vi "motion_server.vi"() -> ()   [LabVIEW 2012]
uses:
  motion_command.ctl
  motion_status.ctl
  <vilib>/Platform/TimedLoop/XDataNode/timing_clust.ctl
  <vilib>/Platform/TimedLoop/XDataNode/nitl_modes.ctl
  <vilib>/Platform/TimedLoop/XDataNode/wakeup.ctl
  <vilib>/Motion/FlexMotion/FunctionsVIs/StartStopMotion.llb/Stop Motion (6 axes).flx
  <vilib>/Platform/TimedLoop/XDataNode/XDataNode.xnode
  <vilib>/Platform/TimedLoop/XDataNode/XDNodeRunTimeDep.lvlib
panel:
  out "Home position":dbl[](array[numeric])
  out "End transform":dbl[](array[numeric])
  in  "Home":bool
  out "Motion status":T1={"Axis names"=["X", "Y", "Z", "Rx", "Ry", "Rz"], "Axis positions"=[], "Pose"=[], "Timestamp"=0, "Ready"=FALSE, "Stopped"=FALSE} {"Pose" format="%#.4f"; "Axis positions" format="%#.4f"}
  out "Stopped":bool
  in  "Emergency stop":bool
  in  "Home found":bool
  out "Command":T2={"Position"=[0.0, 0.0, 0.0, 0.0, 0.0, 0.0], "Axis enable"=[TRUE, TRUE, TRUE, TRUE, TRUE, TRUE], "Mode"=enum."Absolute axis", "Timestamp"=0}
  in  "Set origin":bool
  in  "stop":bool
  # "Motion server"
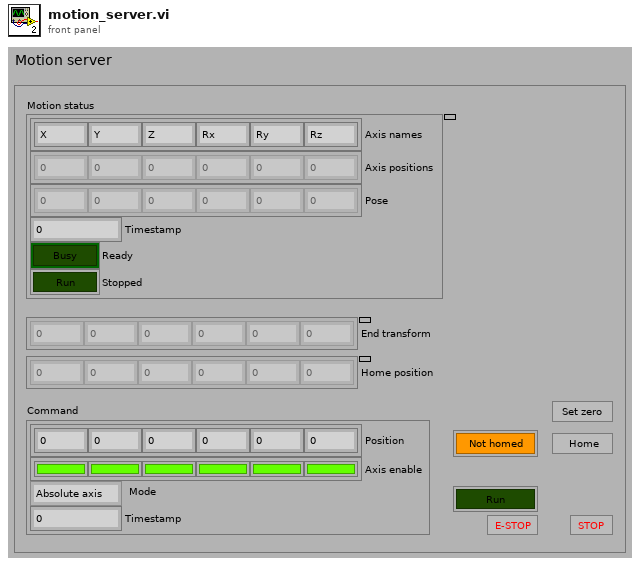
[diagram p1: front panel]
types:
  T1 = typedef "motion_status.ctl" = cluster{"Axis names":string[], "Axis positions":dbl[], "Pose":dbl[], "Timestamp":u32, "Ready":bool, "Stopped":bool}
  T2 = typedef "motion_command.ctl" = cluster{"Position":dbl[], "Axis enable":bool[], "Mode":enum16{"Absolute axis", "Relative axis", "Pose"}, "Timestamp":u32}
  T3 = typedef "Board Id" = u8
  T4 = typedef "Axis #" = cluster{"1":bool, "2":bool, "3":bool, "4":bool, "5":bool, "6":bool}
  T5 = typedef "XDNodeRunTimeDep.lvlib/timing_clust.ctl" = cluster{"Expected End [f-1]":u64, "Actual End [f-1]":u64, "Finished Late? [f-1]":bool, "Expected End [i-1]":u64, "Actual End [i-1]":u64, "Finished Late? [i-1]":bool, "Expected Start [i]":u64, "Actual Start [i]":u64, "Expected Start [f]":u64, "Actual Start [f]":u64, "Source Name":string, "Structure Name":string, "Period":i64, "Deadline":i64, "Offset":i64, "Start":i64, "Priority":i32, "Timeout":i32, "Mode":T6, "Wakeup Reason":T7, "Error":errorcluster, "Source Type":string, "Secondary Source Type":string, "Global End Time":u64, "Global Start Time":u64, "Frame Duration":u64, "Iteration Duration":u64, "Assigned CPU":i32, "I/O Scan Engine Mode":u32}
  T6 = typedef "XDNodeRunTimeDep.lvlib/nitl_modes.ctl" = enum32{"No Change", "Process missed periods, maintain original phase", "Discard missed periods, maintain original phase", "Process missed periods, ignore original phase", "Discard missed periods, ignore original phase"}
  T7 = typedef "XDNodeRunTimeDep.lvlib/wakeup.ctl" = enum32{"Normal", "Aborted", "Asynchronous wakeup", "Timing source error", "Timed loop error", "Timeout"}
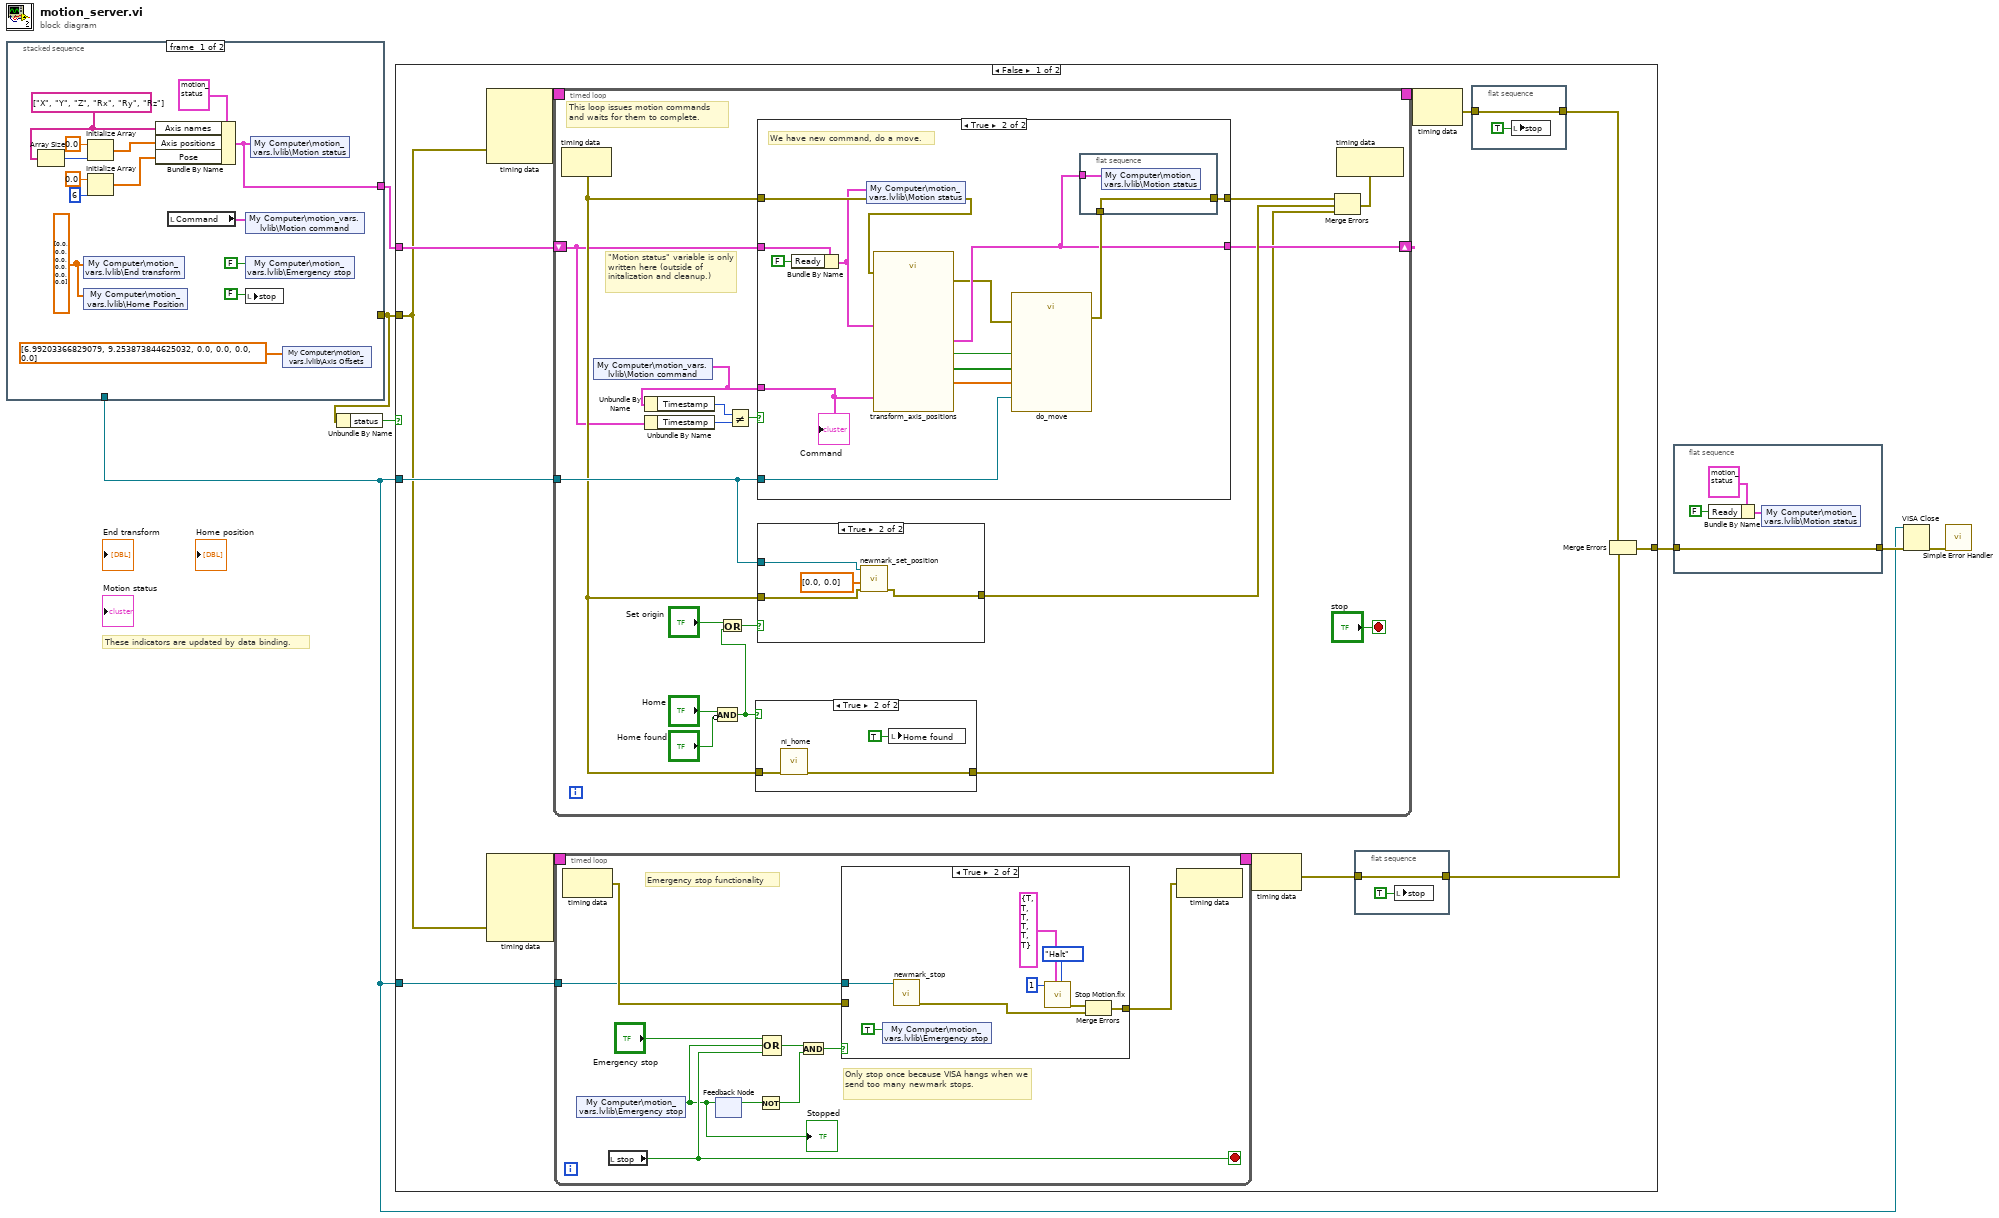
[diagram p0: block diagram]
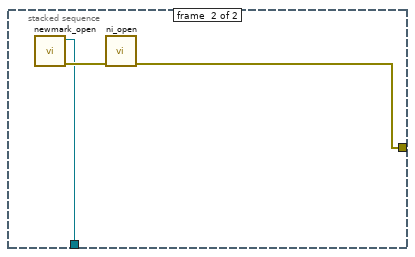
[diagram p2: hidden frame]
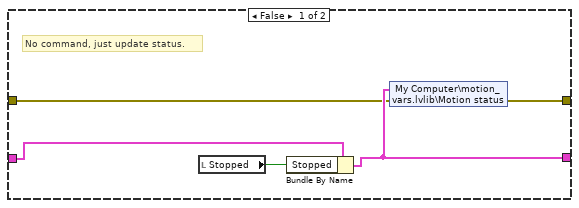
[diagram p6: hidden frame]
diagram:
  # "These indicators are updated by data binding."
  n1 = stacked-sequence {
    tunnel: [_ w22] -> w2
    tunnel: [w10 _] -> w3
    tunnel: [_ w23] -> w1
    frame #0 {
      w11 = string[] ["X", "Y", "Z", "Rx", "Ry", "Rz"] ("Axis names")
      w9 = dbl[] [0.0, 0.0, 0.0, 0.0, 0.0, 0.0] ("End transform")
      n2 = Array Size(array=w11) -> (size(s)=w19:i32)
      n3 = shared-variable "My Computer\\motion_vars.lvlib\\End transform"(w9) -> ()  [unwired: 1 in, 1 out]
      n4 = shared-variable "My Computer\\motion_vars.lvlib\\Home Position"(w9) -> ()  [unwired: 1 in, 1 out]
      n5 = Initialize Array(0.0, w19) -> (w17:dbl[])
      n6 = Initialize Array(0.0, 6 ("dimension size")) -> (w14:dbl[])
      n7 = Bundle By Name(cluster=T1 {"Axis names"=["X", "Y", "Z", "Rx", "Ry", "Rz"], "Axis positions"=[], "Pose"=[], "Timestamp"=0, "Ready"=TRUE, "Stopped"=FALSE} ("Motion status"), "Axis names"=w11, "Axis positions"=w17, "Pose"=w14) -> (w10:T1)
      n8 = local read "Command"() -> (w21:T2)
      n9 = shared-variable "My Computer\\motion_vars.lvlib\\Motion command"(w21) -> ()  [unwired: 1 in, 1 out]
      n10 = shared-variable "My Computer\\motion_vars.lvlib\\Emergency stop"(FALSE ("Emergency stop")) -> ()  [unwired: 1 in, 1 out]
      n11 = local write "stop"(FALSE ("stop")) -> ()
      n12 = shared-variable "My Computer\\motion_vars.lvlib\\Motion status"(w10) -> ()  [unwired: 1 in, 1 out]
      n13 = shared-variable "My Computer\\motion_vars.lvlib\\Axis Offsets"(dbl[] [6.99203366829079, 9.253873844625032, 0.0, 0.0, 0.0, 0.0] ("Axis offsets")) -> ()  [unwired: 1 in, 1 out]
    }
    frame #1 {
      n14 = call "newmark_open.vi"() -> ("error out"=w24:errorcluster, "VISA Refnum out"=w23:refnum<visa-resource-name>)  [unwired: 10 in]
      n15 = call "ni_open.vi"("error in"=w24) -> ("error out"=w22:errorcluster)  [unwired: 10 in]
    }
  }
  n16 = Unbundle By Name(w2) -> ("status"=w7:bool)
  n17 = case shown="False" w7 {
    tunnel: w2 -> [w29 w129]
    tunnel: w1 -> [w33 _]
    tunnel: [w32 w129] -> w5
    tunnel: w3 -> [w31 _]
    tunnel: w1 -> [w30 _]
    frame False {
      n18 = node-c288(w29) -> (w37:T5)  [unwired: 3 in]
      n19 = node-c288(w29) -> (w35:T5)  [unwired: 4 in]
      n20 = timed-loop {
        tunnel: w33 -> [w84]
        timing: w37 -> [_]
        timing-out: [_] -> w36
        shift-right: [w82] -> _
        shift-left: w31 -> [w71]
        stop <- "stop" stop-if-true
        # "\"Motion status\" variable is only written here (outside of initalization and cleanup.)"
        # "This loop issues motion commands\nand waits for them to complete."
        n21 = node-c288() -> (w78:errorcluster)  [unwired: 1 in]
        n22 = shared-variable "My Computer\\motion_vars.lvlib\\Motion command"() -> (w79:T2)  [unwired: 1 in, 1 out]
        n23 = Unbundle By Name(w79) -> ("Timestamp"=w80:u32)
        n24 = Unbundle By Name(w71) -> ("Timestamp"=w81:u32)
        n25 = Compound Arithmetic op=AND("Home", invert "Home found") -> (w72:bool)
        n26 = Or(x="Set origin", y=w72) -> (x .or. y?=w73:bool)
        n27 = Not Equal?(x=w80, y=w81) -> (x != y?=w83:bool)
        n28 = case shown="True" w72 {
          tunnel: w78 -> [w89 w92]
          tunnel: [w89 w91] -> w77
          frame False {
          }
          frame True {
            n29 = call "ni_home.vi"("error in"=w92) -> ("error out"=w91:errorcluster)  [unwired: 10 in]
            n30 = local write "Home found"(TRUE ("Home found")) -> ()
          }
        }
        n31 = case shown="True" w83 {
          tunnel: w84 -> [_ w116]
          tunnel: [w98 w113] -> w87
          tunnel: w71 -> [w102 w115]
          tunnel: [w100 w111] -> w82
          tunnel: w78 -> [w99 w110]
          tunnel: w79 -> [_ w103]
          frame False {
            # "No command, just update status."
            n32 = local read "Stopped"() -> (w101:bool)
            n33 = Bundle By Name(cluster=w102, "Stopped"=w101) -> (w100:T1)
            n34 = shared-variable "My Computer\\motion_vars.lvlib\\Motion status"(w100, error in=w99) -> (error out=w98:errorcluster)
          }
          frame True {
            # "We have new command, do a move."
            n35 = Bundle By Name(cluster=w115, "Ready"=FALSE) -> (w104:T1)
            n36 = shared-variable "My Computer\\motion_vars.lvlib\\Motion status"(w104, error in=w110) -> (error out=w105:errorcluster)
            n37 = call "transform_axis_positions.vi"("Current status"=w104, "error in"=w105, "Command"=w103) -> ("error out"=w106:errorcluster, "Absolute"=w109:bool, "Axis positions"=w107:dbl[], "Axis enable"=w108:bool[], "Final status"=w111:T1)  [unwired: 4 in]
            n38 = call "do_move.vi"("Absolute"=w109, "error in"=w106, "Axis positions"=w107, "Axis enable"=w108, "Newmark handle"=w116) -> ("error out"=w112:errorcluster)  [unwired: 6 in]
            n39 = flat-sequence {
              tunnel: [w117] -> w113
              tunnel: w112 -> [w117]
              tunnel: w111 -> [w118]
              frame #0 {
                n40 = shared-variable "My Computer\\motion_vars.lvlib\\Motion status"(w118) -> ()  [unwired: 1 in, 1 out]
              }
            }
            "Command" <- w103
          }
        }
        n41 = case shown="True" w73 {
          tunnel: w84 -> [_ w97]
          tunnel: w78 -> [w93 w95]
          tunnel: [w93 w94] -> w85
          frame False {
          }
          frame True {
            n42 = call "newmark_set_position.vi"("error in"=w95, "Axis positions"=dbl[] [0.0, 0.0], "VISA Refnum in"=w97) -> ("error out"=w94:errorcluster)  [unwired: 7 in, 1 out]
          }
        }
        n43 = Merge Errors(w87, w85, w77) -> (w86:errorcluster)
        n44 = node-c288(w86) -> ()  [unwired: 1 out]
      }
      n45 = timed-loop {
        timing: w35 -> [_]
        timing-out: [_] -> w34
        tunnel: w30 -> [w49]
        stop <- w47 stop-if-true
        # "Emergency stop functionality"
        # "Only stop once because VISA hangs when we send too many newmark stops."
        n46 = node-c288() -> (w51:errorcluster)  [unwired: 1 in]
        n47 = shared-variable "My Computer\\motion_vars.lvlib\\Emergency stop"() -> (w42:bool)  [unwired: 1 in, 1 out]
        "Stopped" <- w42
        n48 = local read "stop"() -> (w47:bool)
        n49 = feedback-in #1(w42) -> ()
        n50 = feedback #1() -> (w44:bool)  [unwired: 1 in]
        n51 = Not(x=w44) -> (.not. x?=w45:bool)
        n52 = Compound Arithmetic op=OR("Emergency stop", w42, w47) -> (w46:bool)
        n53 = And(x=w46, y=w45) -> (x .and. y?=w43:bool)
        n54 = case shown="True" w43 {
          tunnel: w51 -> [w52 _]
          tunnel: [w52 w55] -> w50
          tunnel: w49 -> [_ w57]
          frame False {
          }
          frame True {
            n55 = shared-variable "My Computer\\motion_vars.lvlib\\Emergency stop"(TRUE ("Emergency stop")) -> ()  [unwired: 1 in, 1 out]
            n56 = call "newmark_stop.vi"("VISA Refnum in"=w57) -> ("error out"=w53:errorcluster)  [unwired: 9 in, 1 out]
            n57 = call-poly <vilib>:"Stop Motion.flx"("Stop Type (Decel)"=enum16{"Decelerate", "Halt", "Kill"}."Halt", "Axis/VS Map"=T4 {"1"=TRUE, "2"=TRUE, "3"=TRUE, "4"=TRUE, "5"=TRUE, "6"=TRUE}, "Board ID"=T3 1) -> ("error out"=w54:errorcluster)  [unwired: 4 in, 2 out]
            n58 = Merge Errors(w54, w53) -> (w55:errorcluster)
          }
        }
        n59 = node-c288(w50) -> ()  [unwired: 1 out]
      }
      n60 = node-c288(w34) -> (w28:errorcluster)
      n61 = flat-sequence {
        tunnel: w28 -> [w40]
        tunnel: [w40] -> w27
        frame #0 {
          n62 = local write "stop"(TRUE ("stop")) -> ()
        }
      }
      n63 = node-c288(w36) -> (w26:errorcluster)
      n64 = flat-sequence {
        tunnel: w26 -> [w38]
        tunnel: [w38] -> w25
        frame #0 {
          n65 = local write "stop"(TRUE ("stop")) -> ()
        }
      }
      n66 = Merge Errors(w25, w27) -> (w32:errorcluster)
    }
    frame True {
    }
  }
  n67 = flat-sequence {
    tunnel: w5 -> [w133]
    tunnel: [w133] -> w4
    frame #0 {
      n68 = Bundle By Name(cluster=T1 {"Axis names"=["X", "Y", "Z", "Rx", "Ry", "Rz"], "Axis positions"=[], "Pose"=[], "Timestamp"=0, "Ready"=FALSE, "Stopped"=FALSE} ("Motion status"), "Ready"=FALSE ("Moving?")) -> (w131:T1)
      n69 = shared-variable "My Computer\\motion_vars.lvlib\\Motion status"(w131) -> ()  [unwired: 1 in, 1 out]
    }
  }
  n70 = VISA Close(VISA resource name=w1, error in (no error)=w4) -> (error out=w6:errorcluster)
  n71 = call <vilib>:"Simple Error Handler.vi"("error in (no error)"=w6) -> ()  [unwired: 4 in, 5 out]
